vi "UI.UserLogin.vi"(11 "路径":path) -> (1 "LoginUnserName":string, 2 "LoginStatus":enum16{"Logout", "LoginUser", "LoginAdmin"}(ring), 3 "OK?":bool)   [LabVIEW 2012, in "Lib_UEL.ATE.lvlib" / "Lib_App.lvlib"]
uses:
  <vilib>/Utility/config.llb/Read Key (String).vi
  <vilib>/Utility/config.llb/Read Key (I32).vi
  Lib_App.lvlib
  <vilib>/Utility/config.llb/NI_LVConfig.lvlib
panel:
  in  "Cancel":bool
  in  "OK":bool
  in  "PassWord:":string
  in  "UserName:":string
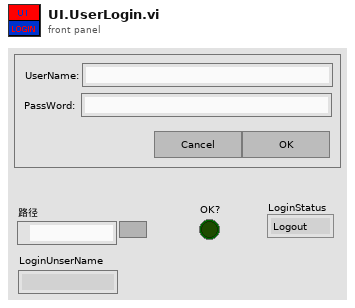
[diagram p1: front panel]
types:
  T1 = typedef "NI_LVConfig.lvlib/Config Data RefNum.ctl" = refnum<k1>
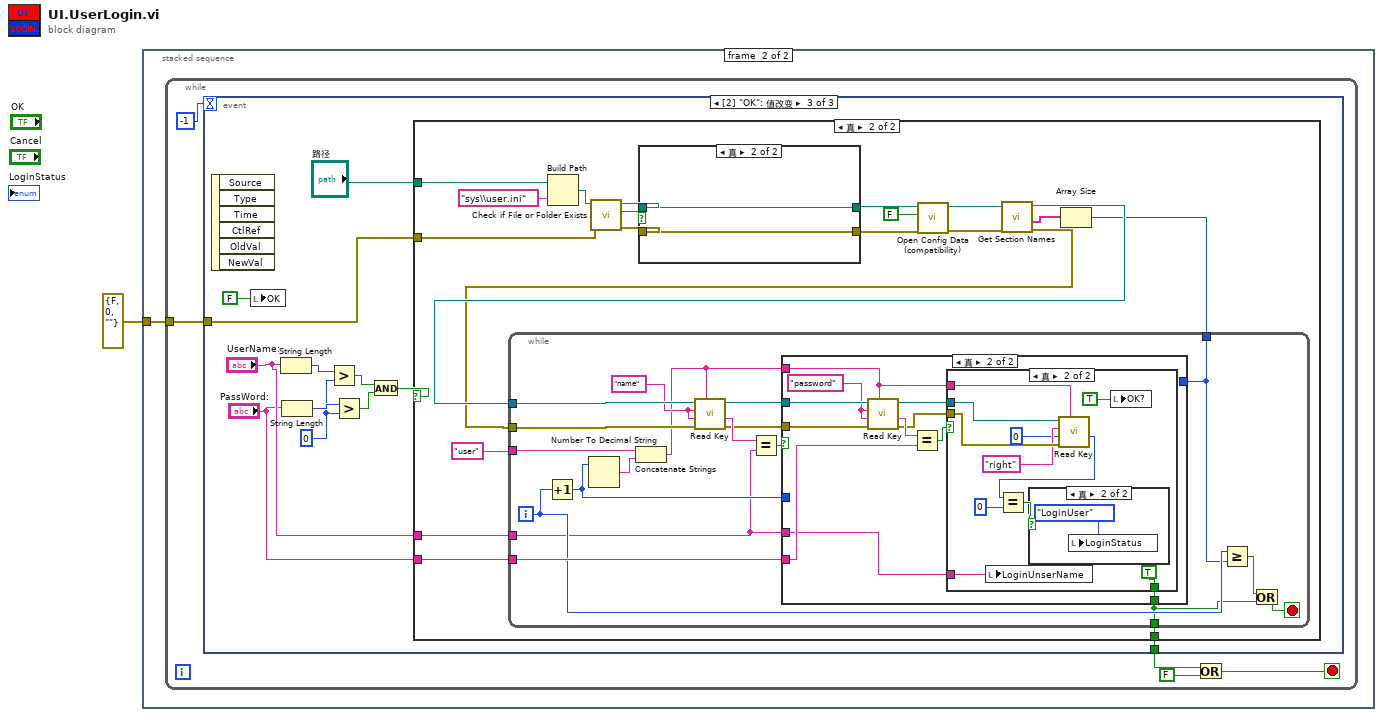
[diagram p0: block diagram]
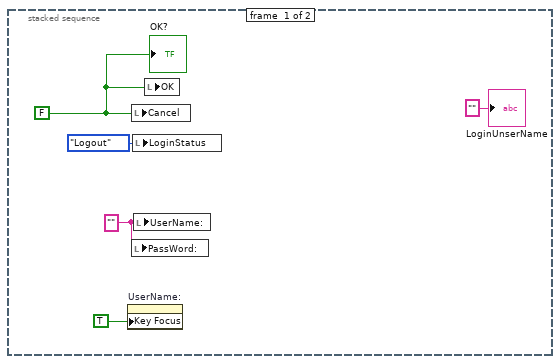
[diagram p2: hidden frame]
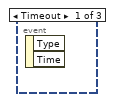
[diagram p3: hidden frame]
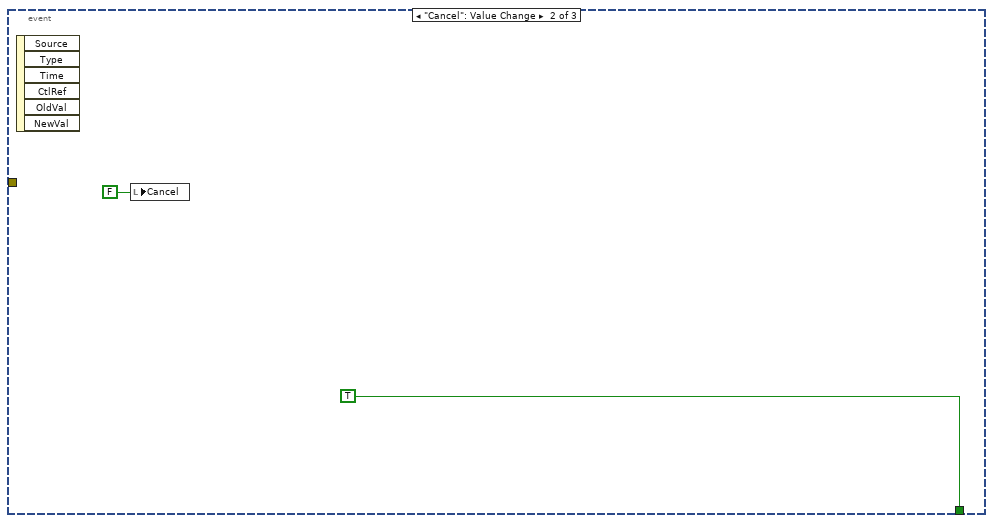
[diagram p4: hidden frame]
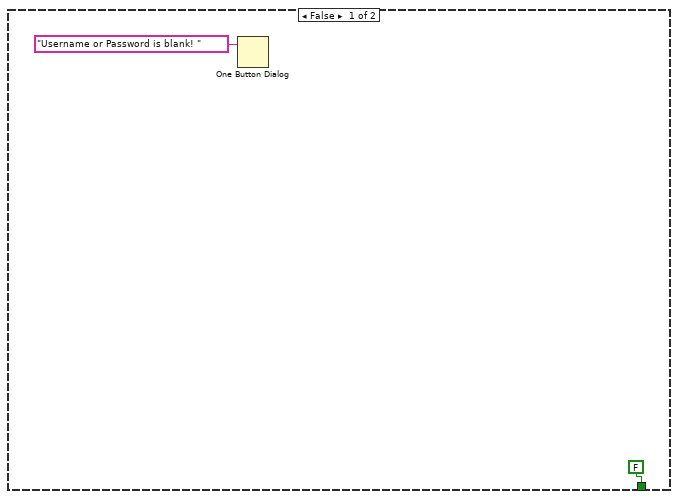
[diagram p5: hidden frame]
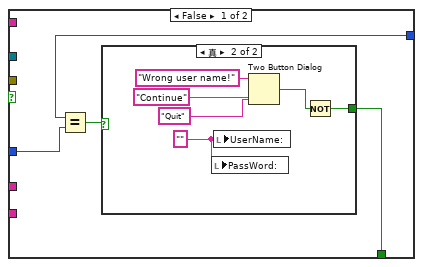
[diagram p6: hidden frame]
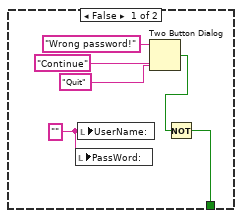
[diagram p8: hidden frame]
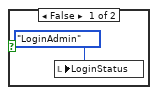
[diagram p9: hidden frame]
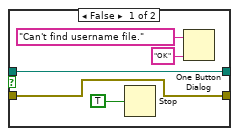
[diagram p10: hidden frame]
diagram:
  n1 = stacked-sequence {
    tunnel: errorcluster {"status"=FALSE, "code"=0, "source"=""} ("error in (no error)") -> [_ w7]
    frame #0 {
      w4 = "" ("UserName:")
      w5 = FALSE ("Cancel")
      n2 = property on="UserName:" class="Str"("Key Focus"=TRUE ("键选中")) -> ()  [unwired: 2 in, 2 out]
      n3 = local write "Cancel"(w5) -> ()
      n4 = local write "PassWord:"(w4) -> ()
      n5 = local write "LoginStatus"(enum16{"Logout", "LoginUser", "LoginAdmin"}."Logout" ("LoginStatus")) -> ()
      n6 = local write "UserName:"(w4) -> ()
      n7 = local write "OK"(w5) -> ()
      "OK?" <- w5
      "LoginUnserName" <- "" ("LoginUnserName")
    }
    frame #1 {
      n8 = while {
        tunnel: w7 -> [w11]
        stop <- w8 stop-if-true
        n9 = event shown="[2] \"OK\": 值改变" {
          selector: _ -> [_ _ _]
          dyn-events: _ -> [_ _ _]
          timeout: -1 -> [_ _ _]
          tunnel: [_ TRUE ("Cancel") w15] -> w10
          tunnel: w11 -> [_ _ w18]
          event Timeout {
            n10 = event-data() -> ()  [unwired: 1 in, 2 out]
          }
          event "Cancel": Value Change {
            n11 = event-data() -> ()  [unwired: 1 in, 6 out]
            n12 = local write "Cancel"(FALSE ("Cancel")) -> ()
          }
          event "OK": Value Change {
            w23 = 0 ("y")
            n13 = event-data() -> ()  [unwired: 1 in, 6 out]
            n14 = local write "OK"(FALSE ("OK")) -> ()
            n15 = String Length(string="UserName:") -> (length=w25:i32)
            n16 = String Length(string="PassWord:") -> (length=w24:i32)
            n17 = Greater?(x=w25, y=w23) -> (0:w22:bool)
            n18 = Greater?(x=w24, y=w23) -> (0:w21:bool)
            n19 = And(x=w22, y=w21) -> (x .and. y?=w20:bool)
            n20 = case shown="真" w20 {
              tunnel: "路径" -> [_ w43]
              tunnel: w18 -> [_ w42]
              tunnel: "UserName:" -> [_ w34]
              tunnel: "PassWord:" -> [_ w33]
              tunnel: [FALSE w30] -> w15
              frame False {
                n21 = One Button Dialog(message="Username or Password is blank! " ("消息")) -> ()  [unwired: 1 in, 1 out]
              }
              frame True {
                n22 = Build Path(base path=w43, name or relative path="sys\\user.ini" ("名称或相对路径")) -> (appended path=w45:path)
                n23 = call <vilib>:"Check if File or Folder Exists.vi"("error in (no error)"=w42, "path"=w45) -> ("error out"=w47:errorcluster, "file or folder exists?"=w46:bool, "dup path"=w48:path)  [unwired: 7 in]
                n24 = case shown="真" w46 {
                  tunnel: w47 -> [w108 w114]
                  tunnel: w48 -> [w109 w113]
                  tunnel: [w108 w114] -> w40
                  tunnel: [w109 w113] -> w41
                  frame False {
                    n25 = Stop(stop? (T)=TRUE ("停止？(T)")) -> ()
                    n26 = One Button Dialog(message="Can't find username file." ("消息"), button name ("OK")="OK" ("按钮名称（“确定”）")) -> ()  [unwired: 1 out]
                  }
                  frame True {
                  }
                }
                n27 = call <vilib>:"Open Config Data (compatibility).vi"("error in (no error)"=w40, "create file if necessary (T)"=FALSE ("create file if necessary? (T)"), "configuration file path"=w41) -> ("error out"=w37:errorcluster, "refnum"=w38:T1)  [unwired: 6 in, 1 out]
                n28 = call <vilib>:"Get Section Names.vi"("error in (no error)"=w37, "refnum"=w38) -> ("error out"=w35:errorcluster, "section names"=w32:string[], "refnum out"=w36:T1)  [unwired: 7 in]
                n29 = Array Size(array=w32) -> (size(s)=w29:i32)
                n30 = while {
                  tunnel: "user" ("名称或相对路径") -> [w66]
                  tunnel: w36 -> [w64]
                  tunnel: w35 -> [w63]
                  tunnel: w34 -> [w49]
                  tunnel: w33 -> [w56]
                  tunnel: [w53] -> w30
                  tunnel: w29 -> [w51]
                  i -> [w54]
                  stop <- w52 stop-if-true
                  w62 = "name" ("key")
                  n31 = Increment(x=w54) -> (x+1=w50:i32)
                  n32 = Number To Decimal String(number=w50) -> (decimal integer string=w65:string)  [unwired: 1 in]
                  n33 = Concatenate Strings(w66, w65) -> (w59:string)
                  n34 = call-poly <vilib>:"Read Key.vi"("section"=w59, "error in (no error)"=w63, "default value"=w62, "key"=w62, "refnum"=w64) -> ("error out"=w57:errorcluster, "value"=w61:string, "refnum out"=w58:T1)  [unwired: 3 in, 1 out]
                  n35 = Equal?(x=w61, y=w49) -> (x = y?=w60:bool)
                  n36 = case shown="真" w60 {
                    tunnel: w59 -> [_ w82]
                    tunnel: w58 -> [_ w88]
                    tunnel: w57 -> [_ w87]
                    tunnel: w56 -> [_ w84]
                    tunnel: [w70 w79] -> w53
                    tunnel: w51 -> [w68 _]
                    tunnel: w50 -> [w67 _]
                    tunnel: w49 -> [_ w78]
                    frame False {
                      n37 = Equal?(x=w68, y=w67) -> (x = y?=w69:bool)
                      n38 = case shown="真" w69 {
                        selector: w69 -> [w71 _]
                        tunnel: [w71 w73] -> w70
                        frame False {
                        }
                        frame True {
                          w72 = "" ("UserName:")
                          n39 = local write "PassWord:"(w72) -> ()
                          n40 = local write "UserName:"(w72) -> ()
                          n41 = Two Button Dialog(message="Wrong user name!" ("消息"), 1:"Quit" ("T按钮名称（“确定”）"), 2:"Continue" ("T按钮名称（“确定”）")) -> (T button?=w74:bool)
                          n42 = Not(x=w74) -> (.not. x?=w73:bool)
                        }
                      }
                    }
                    frame True {
                      w86 = "password" ("key")
                      n43 = call-poly <vilib>:"Read Key.vi"("section"=w82, "error in (no error)"=w87, "default value"=w86, "key"=w86, "refnum"=w88) -> ("error out"=w80:errorcluster, "value"=w85:string, "refnum out"=w81:T1)  [unwired: 3 in, 1 out]
                      n44 = Equal?(x=w85, y=w84) -> (x = y?=w83:bool)
                      n45 = case shown="真" w83 {
                        tunnel: w82 -> [_ w105]
                        tunnel: w81 -> [_ w104]
                        tunnel: w80 -> [_ w103]
                        tunnel: [w90 TRUE] -> w79
                        tunnel: w78 -> [_ w95]
                        frame False {
                          w89 = "" ("UserName:")
                          n46 = local write "PassWord:"(w89) -> ()
                          n47 = local write "UserName:"(w89) -> ()
                          n48 = Two Button Dialog(message="Wrong password!" ("消息"), 1:"Quit" ("T按钮名称（“确定”）"), 2:"Continue" ("T按钮名称（“确定”）")) -> (T button?=w91:bool)
                          n49 = Not(x=w91) -> (.not. x?=w90:bool)
                        }
                        frame True {
                          n50 = local write "LoginUnserName"(w95) -> ()
                          n51 = call-poly <vilib>:"Read Key.vi"("section"=w105, "error in (no error)"=w103, "default value"=0, "key"="right", "refnum"=w104) -> ("value"=w100:i32)  [unwired: 3 in, 3 out]
                          n52 = Equal?(x=w100, y=0) -> (x = y?=w98:bool)
                          n53 = case shown="真" w98 {
                            frame False {
                              n54 = local write "LoginStatus"(enum16{"Logout", "LoginUser", "LoginAdmin"}."LoginAdmin" ("LoginStatus")) -> ()
                            }
                            frame True {
                              n55 = local write "LoginStatus"(enum16{"Logout", "LoginUser", "LoginAdmin"}."LoginUser" ("LoginStatus")) -> ()
                            }
                          }
                          n56 = local write "OK?"(TRUE ("OK?")) -> ()
                        }
                      }
                    }
                  }
                  n57 = Greater Or Equal?(x=w54, y=w51) -> (x >= y?=w55:bool)
                  n58 = Or(x=w55, y=w53) -> (x .or. y?=w52:bool)
                }
              }
            }
          }
        }
        n59 = Or(x=w10, y=FALSE) -> (x .or. y?=w8:bool)
      }
    }
  }
